vi "RSZVB Get Slope.vi"(8 "error in (no error)":errorcluster {"code" format="%.0x"}, 9 "Port (1)":i32=1, 10 "Channel (1)":i32=1, 11 "VISA session":refnum<visa-resource-name>) -> (0 "error out":errorcluster {"code" format="%.0x"}, 2 "Slope":dbl format="%^.3e", 3 "dup VISA session":refnum<visa-resource-name>)   [LabVIEW 2011]
doc: "This VI returns a linear factor to modify the internal source power at port <Pt> as a VI of the stimulus frequency. \n\nNote(s):\n\n(1) The value can be set for frequency sweeps only.\n\nRemote-control command(s):\nSOURce<Ch>:POWer<Pt>[:LEVel][:IMMediate]:SLOPe?"
uses:
  _utility/RSZVB Global Data.vi
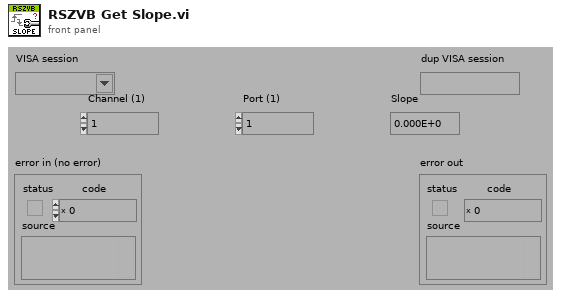
[diagram p1: front panel]
types:
  T1 = cluster{"Error Checking (T: On)":bool, "Installed Options":string[], "Data Valid?":bool, "Ports":i32, "Model":string[], "Option Checking (T: On)":bool}[]
  T2 = cluster{"Error Checking (T: On)":bool, "Installed Options":string[], "Data Valid?":bool, "Ports":i32, "Model":string[], "Option Checking (T: On)":bool}
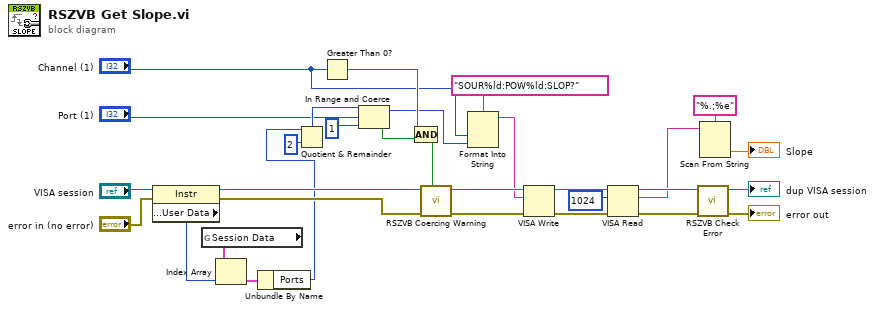
[diagram p0: block diagram]
diagram:
  n1 = property class="Instr"(reference="VISA session", error in="error in (no error)") -> (reference out=w21:refnum<visa-resource-name>, error out=w22:errorcluster, "General Settings:User Data"=w23:u32)
  n2 = global read "RSZVB Global Data.vi" "Session Data"() -> (w24:T1)
  n3 = Index Array(array=w24, index=w23) -> (element=w25:T2)
  n4 = Unbundle By Name(w25) -> ("Ports"=w15:i32)
  n5 = Quotient & Remainder(x=w15, y=2) -> (floor(x/y)=w17:i32)  [unwired: 1 out]
  n6 = Greater Than 0?(x="Channel (1)") -> (x > 0?=w26:bool)
  n7 = In Range and Coerce(upper limit=w17, x="Port (1)", lower limit=1) -> (coerced(x)=w16:i32, In Range?=w19:bool)
  n8 = Compound Arithmetic op=AND(w26, w19) -> (w28:bool)
  n9 = call "RSZVB Coercing Warning.vi"("In Range?"=w28, "error in (no error)"=w22, "VISA session"=w21) -> ("error out"=w29:errorcluster, "dup VISA session"=w30:refnum<visa-resource-name>)  [unwired: 7 in]
  n10 = Format Into String(format string="SOUR%ld:POW%ld:SLOP?", "Channel (1)", w16) -> (resulting string=w27:string)  [unwired: 2 in, 1 out]
  n11 = VISA Write(VISA resource name=w30, write buffer=w27, error in (no error)=w29) -> (VISA resource name out=w6:refnum<visa-resource-name>, error out=w7:errorcluster)  [unwired: 1 out]
  n12 = VISA Read(VISA resource name=w6, byte count=u32 1024 ("byte count (0)"), error in (no error)=w7) -> (VISA resource name out=w9:refnum<visa-resource-name>, read buffer=w1:string, error out=w8:errorcluster)  [unwired: 1 out]
  n13 = call "RSZVB Check Error.vi"("error in (no error)"=w8, "VISA session"=w9) -> ("error out"=→"error out":errorcluster, "dup VISA session"=→"dup VISA session":refnum<visa-resource-name>)  [unwired: 8 in]
  n14 = Scan From String(format string="%.;%e", input string=w1) -> (output 1=→"Slope":dbl)  [unwired: 3 in, 3 out]
